vi "Count Num of True Element in 2D Array.vi"(8 "错误输入":errorcluster, 10 "Mode":enum16{"Row", "Col"}(ring), 11 "2D Boolean Array":bool[][](array[boolean])) -> (0 "错误输出":errorcluster, 3 "Num of True":i16[](array[numeric]))   [LabVIEW 2012]
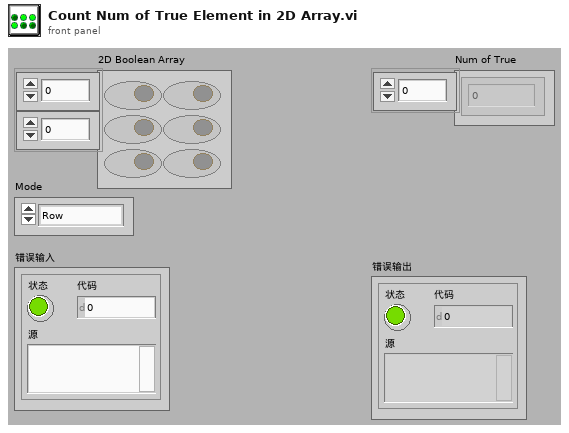
[diagram p1: front panel]
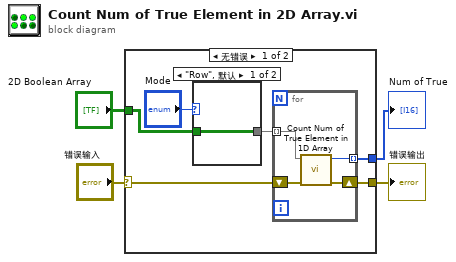
[diagram p0: block diagram]
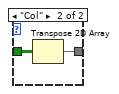
[diagram p2: hidden frame]
diagram:
  n1 = case shown="无错误" "错误输入" {
    selector: "错误输入" -> [w7 w18]
    tunnel: [w5 w18] -> w3
    tunnel: "2D Boolean Array" -> [w9 _]
    tunnel: [w6 _] -> w1
    frame No Error {
      n2 = case shown="\"Row\", 默认" "Mode" {
        tunnel: w9 -> [w15 w17]
        tunnel: [w15 w16] -> w8
        frame "Row", Default {
        }
        frame "Col" {
          n3 = Transpose 2D Array(2D array=w17) -> (transposed array=w16:bool[][])
        }
      }
      n4 = for {
        tunnel: w8 -> [w14] mode=indexing
        shift-right: [w12] -> w5
        shift-left: w7 -> [w13]
        tunnel: [w11] -> w6 mode=indexing
        n5 = call "Count Num of True Element in 1D Array.vi"("错误输入"=w13, "Boolean Array(1D)"=w14) -> ("错误输出"=w12:errorcluster, "Num of True"=w11:i16)  [unwired: 8 in]
      }
    }
    frame Error {
    }
  }
  "Num of True" <- w1
  "错误输出" <- w3
